vi "Lambda_Guide-plot.vi"(6 "Time In":i32, 8 "Temperature Sync":i32, 9 "Temp Band % (e.g. 1%=1.01)":dbl=1.04, 10 "Mean(Off)/Interval(On)":bool, 11 "Guide":bool) -> (2 "Graph 2":dbl, 3 "Graph 1":dbl, 4 "Time out":i32)   [LabVIEW 2014]
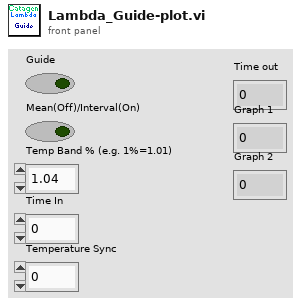
[diagram p1: front panel]
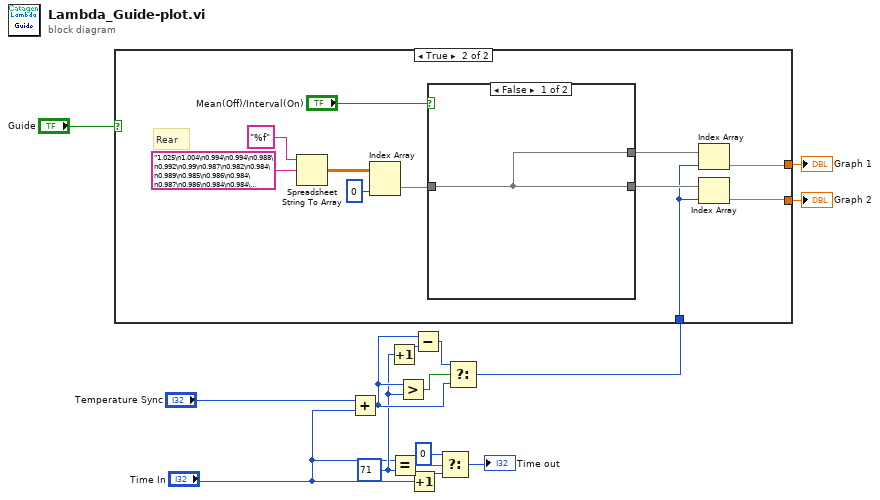
[diagram p0: block diagram]
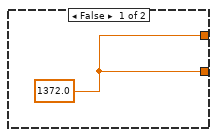
[diagram p2: hidden frame]
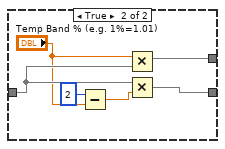
[diagram p3: hidden frame]
diagram:
  w6 = 71 ("y")
  n1 = Add(x="Temperature Sync", y="Time In") -> (x+y=w8:i32)
  n2 = Increment(x=w6) -> (x+1=w7:i32)
  n3 = Equal?(x="Time In", y=w6) -> (x = y?=w13:bool)
  n4 = Greater?(x=w8, y=w6) -> (0:w10:bool)
  n5 = Increment(x="Time In") -> (x+1=w11:i32)
  n6 = Subtract(x=w8, y=w7) -> (x-y=w9:i32)
  n7 = Select(t=0, s=w13, f=w11) -> (s? t:f=→"Time out":i32)
  n8 = Select(t=w9, s=w10, f=w8) -> (s? t:f=w5:i32)
  n9 = case shown="True" "Guide" {
    tunnel: w5 -> [_ w17]
    tunnel: [w16 w18] -> w2
    tunnel: [w16 w19] -> w1
    frame False {
      w16 = 1372.0
    }
    frame True {
      # "Rear"
      n10 = Spreadsheet String To Array(format string="%f", spreadsheet string="1.025\n1.004\n0.994\n0.994\n0.988\n0.992\n0.99\n0.987\n0.982\n0.984\n0.989\n0.985\n0.986\n0.984\n0.987\n0.986\n0.984\n0.984\n0.983\n0.987\n0.986\n0.987\n0.986\n0.986\n0.987\n0.986\n0.987\n1.005\n1.237\n1.238\n1.238\n1.238\n1.238\n1.236\n1.237\n1.064\n0.989\n0.973\n0.984\n0.99\n0.989\n0.989\n0.989\n0.989\n0.989\n0.987\n0.987\n0.986\n0.987\n0.987\n0.986\n0.986\n0.983\n0.984\n0.986\n0.983\n0.983\n0.984\n0.984\n0.983\n0.984\n0.984\n0.995\n1.14\n1.237\n1.237\n1.237\n1.237\n1.237\n1.237\n1.237\n1.135") -> (array=w25:dbl[][])  [unwired: 2 in]
      n11 = Index Array(array=w25, index (col)=0 ("disabled index (col)")) -> (element=w23:dbl[])  [unwired: 1 in]
      n12 = case shown="False" "Mean(Off)/Interval(On)" {
        tunnel: w23 -> [w28 w31]
        tunnel: [w28 w32] -> w21
        tunnel: [w28 w33] -> w20
        frame False {
        }
        frame True {
          n13 = Subtract(x=2, y="Temp Band % (e.g. 1%=1.01)") -> (x-y=w29:dbl)
          n14 = Multiply(x="Temp Band % (e.g. 1%=1.01)", y=w31) -> (x*y=w33:dbl[])
          n15 = Multiply(x=w31, y=w29) -> (x*y=w32:dbl[])
        }
      }
      n16 = Index Array(array=w20, index=w17) -> (element=w18:dbl)
      n17 = Index Array(array=w21, index=w17) -> (element=w19:dbl)
    }
  }
  "Graph 1" <- w2
  "Graph 2" <- w1
